vi "sm125_acquire.vi"(0 "address":string="10.0.0.212", 2 "open and close":bool=TRUE, 4 "connection ID":refnum<k5>, 5 "linear fit (PD)":bool) -> (14 "Output graph":cluster{dbl[], dbl[]}[](graph), 17 "Main Cluster":T1={"HeaderSize"=20, "Version"=1, "nChannels"=4, "freshestDut"=15, "counter"=4086}, 18 "counter":u32=4086, 19 "WvlIncrement":dbl=0.005)   [LabVIEW 2009]
uses:
  <vilib>/Analysis/NI_AALPro.lvlib
panel:
  in  "remote port":u16=50000
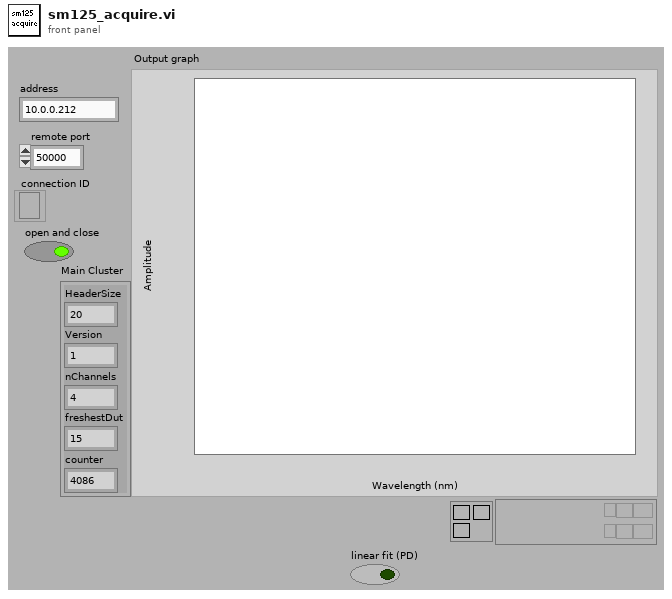
[diagram p1: front panel]
types:
  T1 = cluster{"HeaderSize":u16, "Version":u16, "nChannels":u16, "freshestDut":u16, "counter":u16}
  T2 = cluster{"HeaderSize":u16, "Version":u16, "nChannels":u16, "freshestDut":u16, "counter":i32}
  T3 = cluster{"HeaderSize":u16, "MinWvl":dbl, "WvlIncrement":dbl, "nPoints":u16, "DUT":u16}
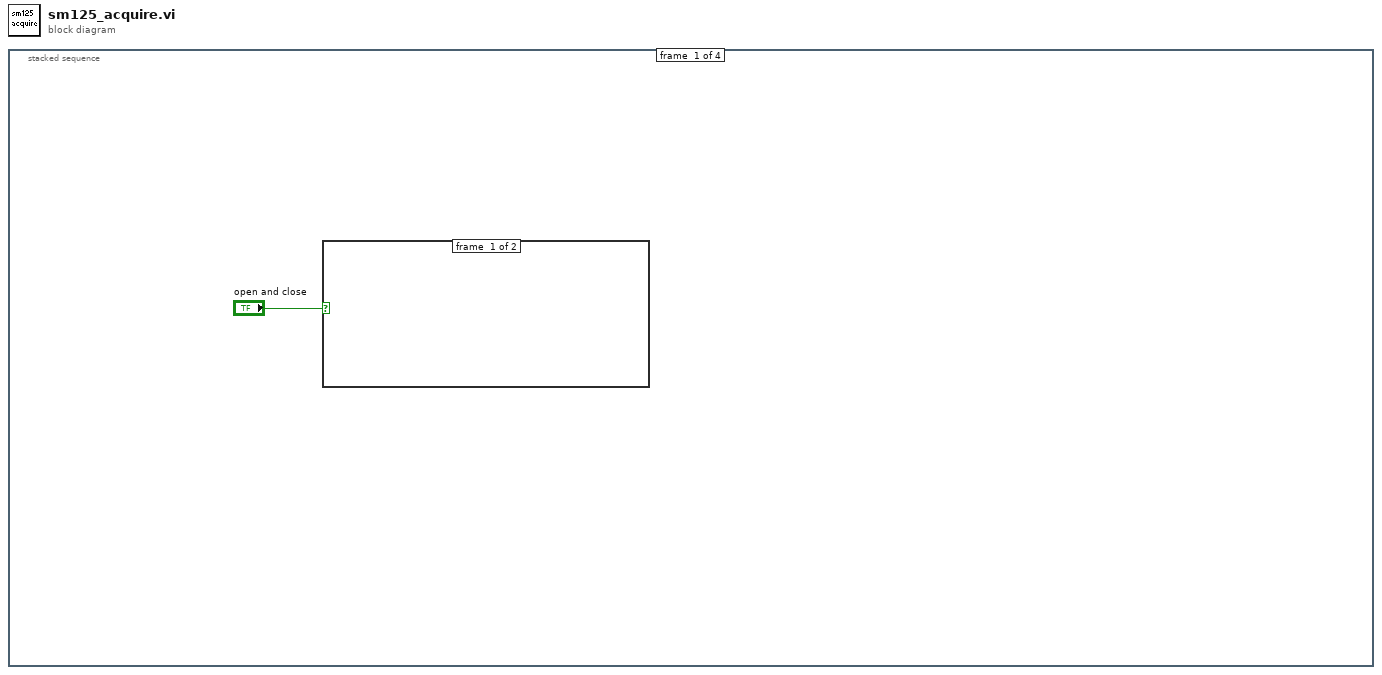
[diagram p0: block diagram]
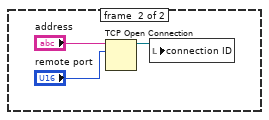
[diagram p2: hidden frame]
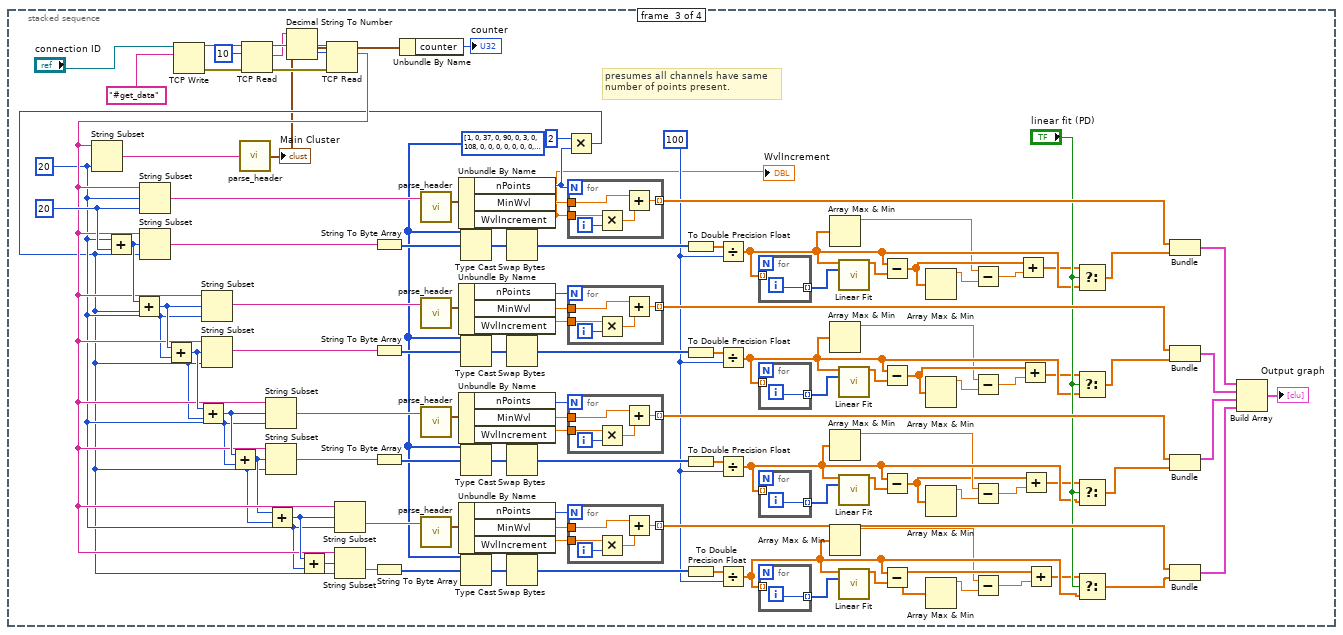
[diagram p4: hidden frame]
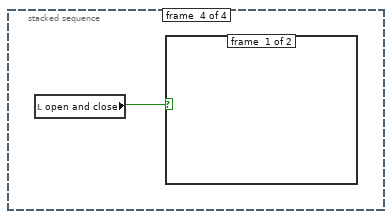
[diagram p5: hidden frame]
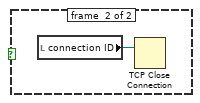
[diagram p6: hidden frame]
diagram:
  n1 = stacked-sequence {
    frame #0 {
      n2 = case shown="True" "open and close" {
        frame #0 {
        }
        frame #1 {
          n3 = TCP Open Connection(address="address", remote port or service name="remote port") -> (connection ID=w4:refnum<k5>)  [unwired: 3 in, 1 out]
          n4 = local write "connection ID"(w4) -> ()
        }
      }
    }
    frame #1 {
    }
    frame #2 {
      w56 = 100
      w57 = i16[] [1, 0, 37, 0, 90, 0, 3, 0, 108, 0, 0, 0, 0, 0, 0, 0, 0, 0, 0, 0, 0, 0, 0, 0, 0, 0, 0, 0, 0, 0, 0, 0, 0, 0, 0, 0, 0, 0, 0, 0, 0, 0, 0, 0, 0, 0, 0, 0, 0, 0, 0, 0, 0, 0, 0, 0, 0, 0, 0, 0, 0, 0, 0, 0, 32, 0, 14, 152, 140, 62, 252, 150, 1, 0, 76, 78, 0, 0, 0, 0, 0, 0, 0, 0, 0, 0, 12, 0, 0, 0, 0, 0, 0, 0, 0, 0, 0, 0, 0, 0, 0, 0, 0, 0, 0, 0, 0, 0, 0, 0, 0, 0, 0, 0, 0, 0, 0, 0, 0, 0, 0, 0, 0, 0, 0, 0, 0, 0, 92, 121, 255, 255, 0, 0, 0, 0, 0, 0, 0, 0, 0, 0, 0, 0, 0, 0, 0, 0, 0, 0, 0, 0, 0, 0, 0, 0, 0, 0, 0, 0, 0, 0, 0, 0, 0, 0, 0, 0, 0, 0, 0, 0, 0, 0, 0, 0, 0, 0, 0, 0, 0, 0, 0, 0, 0, 0, 0, 0, 0, 0, 0, 0, 82, 0, 0, 0, 0, 0, 0, 0, 0, 0, 0, 0, 0, 0, 0, 0, 0, 0, 0, 0, 0, 0, 0, 0, 0, 0, 0, 0, 0, 0, 0, 0, 0, 0, 0, 0, 0, 0, 0, 0, 0, 0, 0, 0, 0, 0, 0, 0, 0, 0, 0, 0, 0, 0, 0, 0, 0, 0, 0, 0, 0, 0, 0, 0, 110, 0, 252, 3, 183, 4, 161, 5, 181, 6, 108, 8, 117, 9, 72, 12, 25, 13, 221, 13, 76, 14, 153, 18, 218, 22, 1, 27, 14, 31, 36, 35, 56, 39, 95, 43, 152, 47, 196, 51, 8, 56, 77, 60, 162, 64, 4, 69, 115, 73, 246, 77, 121, 82, 16, 87, 171, 91, 87, 96, 4, 101, 201, 105, 146, 110, 64, 115, 24, 120, 252, 124, 229, 129, 255, 255, 255, 255, 0, 0, 0, 0, 0, 0, 0, 0, 0, 0, 0, 0, 0, 0, 0, 0, 0, 0, 0, 0, 0, 0, 0, 0, 0, 0, 0, 0, 0, 0, 0, 0, 0, 0, 0, 0, 0, 0, 0, 0, 0, 0, 0, 0, 0, 0, 0, 0, 0, 0, 0, 0, 0, 0, 0, 0, 0, 0, 0, 0, 0, 0, 0, 0, 0, 0, 0, 0, 0, 0, 0, 0, 0, 0, 0, 0, 0, 0, 0, 0, 0, 0, 0, 0, 0, 0, 0, 0, 0, 0, 0, 0, 0, 0, 0, 0, 0, 0, 0, 0, 0, 0, 0, 0, 0, 0, 0, 0, 0, 0, 0, 0, 0, 0, 0, 0, 0, 0, 0, 0, 0, 0, 0, 0, 0, 0, 0, 0, 0, 0, 0, 0, 0, 0, 0, 0, 0, 0, 0, 0, 0, 0, 0, 0, 0, 0, 0, 0, 0, 0, 0, 0, 0, 0, 0, 0, 0, 0, 0, 0, 0, 0, 0, 0, 0, 0, 0, 0, 0, 0, 0, 0, 0, 0, 0, 0, 0, 0, 77, 2, 234, 3, 164, 4, 145, 5, 168, 6, 113, 8, 131, 9, 129, 10, 107, 11, 67, 12, 5, 13, 189, 13, 109, 14, 21, 15, 205, 15, 129, 16, 33, 17, 195, 17, 99, 18, 243, 18, 151, 19, 9, 21, 154, 21, 45, 22, 192, 22, 95, 23, 190, 25, 152, 26, 155, 27, 181, 29, 50, 30, 3, 32, 38, 34, 247, 34, 253, 37, 135, 38, 249, 38, 146, 39, 127, 42, 48, 43, 60, 44, 197, 44, 47, 47, 185, 47, 72, 48, 208, 48, 210, 50, 86, 51, 195, 51, 145, 55, 36, 56, 164, 56, 102, 57, 18, 60, 129, 60, 3, 62, 120, 62, 180, 63, 168, 68, 133, 69, 106, 70, 98, 73, 82, 74, 61, 78, 7, 83, 195, 83, 164, 84, 153, 87, 25, 88, 98, 92, 90, 93, 7, 94, 3, 97, 243, 97, 220, 98, 204, 101, 186, 102, 177, 103, 182, 106, 169, 107, 84, 108, 49, 112, 149, 117, 33, 122, 22, 127, 182, 133, 240, 137, 245, 142, 47, 147, 54, 152, 255, 255, 235, 151, 199, 152, 204, 153, 155, 157, 80, 158, 190, 158, 255, 255, 255, 255, 255, 255, 31, 158, 218, 158, 255, 255, 153, 157, 255, 255, 255, 255, 255, 255, 207, 158, 238, 161, 214, 162, 255, 255, 255, 255, 0, 0, 0, 0, 0, 0, 0, 0, 0, 0, 0, 0, 0, 0, 0, 0, 0, 0, 0, 0, 0, 0, 0, 0, 0, 0, 0, 0, 0, 0, 0, 0, 59, 40, 239, 82, 166, 129, 255, 255, 255, 255, 0, 0, 0, 0, 0, 0, 0, 0, 0, 0, 0, 0, 0, 0, 0, 0, 0, 0, 0, 0, 0, 0, 0, 0, 0, 0, 0, 0, 0, 0, 0, 0, 0, 0, 0, 0, 0, 0, 0, 0, 0, 0, 0, 0, 0, 0, 0, 0, 0, 0, 0, 0, 0, 0, 0, 0, 0, 0, 0, 0, 0, 0, 0, 0, 0, 0, 0, 0, 0, 0, 0, 0, 0, 0, 0, 0, 0, 0, 0, 0, 0, 0, 0, 0, 0, 0, 0, 0, 0, 0, 0, 0, 0, 0, 0, 0, 0, 0, 0, 0, 0, 0, 0, 0, 0, 0, 0, 0, 0, 0, 0, 0, 0, 0, 0, 0, 0, 0, 0, 0, 0, 0, 0, 0, 0, 0, 0, 0, 0, 0, 0, 0, 0, 0, 0, 0, 0, 0, 0, 0, 0, 0, 0, 0, 0, 0, 0, 0, 0, 0, 0, 0, 0, 0, 0, 0, 0, 0, 0, 0, 0, 0, 0, 0, 0, 0, 0, 0, 0, 0, 0, 0, 0, 0, 0, 0, 0, 0, 0, 0, 0, 0, 0, 0, 0, 0, 0, 0, 0, 0, 0, 0, 0, 0, 0, 0, 0, 0, 0, 0, 0, 0, 0, 0, 0, 0, 0, 0, 0, 0, 0, 0, 0, 0, 0, 0, 0, 0, 0, 0, 0, 0, 0, 0, 0, 0, 0, 0, 0, 0, 0, 0, 0, 0, 0, 0, 0, 0, 0, 0, 0, 0, 0, 0, 0, 0, 93, 2, 12, 3, 214, 3, 152, 4, 117, 8, 137, 9, 122, 10, 102, 11, 66, 12, 4, 13, 150, 13, 121, 14, 37, 15, 205, 15, 115, 16, 26, 17, 188, 17, 24, 19, 180, 19, 74, 20, 224, 20, 132, 21, 36, 24, 168, 24, 50, 25, 169, 25, 173, 27, 103, 28, 159, 31, 16, 32, 149, 32, 22, 33, 165, 33, 247, 35, 131, 36, 236, 36, 173, 39, 96, 40, 209, 40, 98, 41, 205, 43, 66, 44, 208, 44, 92, 45, 197, 47, 76, 48, 213, 48, 208, 51, 150, 52, 172, 53, 164, 55, 42, 56, 165, 56, 112, 57, 127, 60, 4, 62, 26, 63, 248, 63, 125, 64, 227, 64, 189, 65, 127, 66, 123, 67, 235, 67, 157, 68, 121, 69, 82, 73, 77, 74, 78, 77, 44, 78, 254, 81, 254, 82, 173, 83, 16, 86, 188, 86, 139, 87, 139, 90, 101, 91, 57, 92, 248, 94, 251, 95, 234, 96, 239, 99, 215, 100, 181, 101, 215, 103, 190, 104, 163, 105, 176, 108, 148, 109, 83, 110, 104, 111, 84, 112, 135, 118, 18, 124, 238, 128, 217, 133, 20, 138, 246, 142, 17, 147, 41, 152, 199, 157, 215, 161, 39, 168, 182, 171, 55, 177, 245, 181, 75, 186, 255, 255, 7, 147, 150, 147, 226, 151, 195, 152, 194, 153, 207, 156, 140, 157, 75, 158, 76, 161, 202, 161, 172, 162, 190, 165, 153, 166, 148, 167, 134, 170, 68, 171, 25, 172, 10, 173, 39, 175, 255, 255, 0, 0, 0, 0, 0, 0, 0, 0, 0, 0, 0, 0, 0, 0, 0, 0, 0, 0, 0, 0, 0, 0, 0, 0, 0, 0, 0, 0, 0, 0, 0, 0, 0, 0, 0, 0, 0, 0, 0, 0, 0, 0, 0, 0, 0, 0, 0, 0, 0, 0, 0, 0, 0, 0, 0, 0, 0, 0, 0, 0, 0, 0, 0, 0, 0, 0, 0, 0, 0, 0, 0, 0, 0, 0, 0, 0, 0, 0, 0, 0, 0, 0, 0, 0, 0, 0, 0, 0, 0, 0, 0, 0, 0, 0, 0, 0, 0, 0, 0, 0, 0, 0, 0, 0, 0, 0, 0, 0, 0, 0, 0, 0, 0, 0, 0, 0, 0, 0, 0, 0, 0, 0, 0, 0, 0, 0, 0, 0, 0, 0, 0, 0, 0, 0, 0, 0, 0, 0, 0, 0, 0, 0, 0, 0, 0, 0, 0, 0, 0, 0, 0, 0, 0, 0, 0, 0, 0, 0, 0, 0, 0, 0, 0, 0, 0, 0, 0, 0, 0, 0, 0, 0, 0, 0, 0, 0, 0, 0, 0, 0, 0, 0, 0, 0, 0, 0, 0, 0, 0, 0, 0, 0, 0, 0, 0, 0, 0, 0, 0, 0, 0, 0, 0, 0, 0, 0, 0, 0, 0, 0, 0, 0, 0, 0, 0, 0, 0, 0, 0, 0, 0, 0, 0, 0, 0, 0, 0, 0, 0, 0, 0, 0, 0, 0, 0, 0, 0, 0, 0, 0, 0, 0, 0, 0, 0, 0, 0, 0, 0, 0, 0, 0, 0, 0, 85, 33, 129, 181, 194, 126, 33, 18, 52, 165, 153, 175, 177, 188, 188, 185, 180, 190, 184, 197, 191, 183, 183, 189, 186, 184, 186, 190, 190, 196, 193, 198, 199, 203, 201, 204, 203, 203, 0, 0, 0, 0, 0, 0, 0, 0, 0, 0, 0, 0, 0, 0, 0, 0, 0, 0, 0, 0, 0, 0, 0, 0, 0, 0, 0, 0, 0, 0, 0, 0, 0, 0, 0, 0, 0, 0, 0, 0, 0, 0, 0, 0, 0, 0, 0, 0, 0, 0, 0, 0, 0, 0, 0, 0, 0, 0, 0, 0, 0, 0, 0, 0, 0, 0, 0, 0, 0, 0, 0, 0, 0, 0, 0, 0, 0, 0, 0, 0, 0, 0, 0, 0, 0, 0, 0, 0, 0, 0, 65, 98, 149, 164, 162, 138, 125, 53, 132, 142, 148, 153, 154, 141, 81, 134, 124, 136, 116, 127, 89, 107, 106, 121, 121, 94, 101, 86, 96, 79, 103, 99, 105, 96, 88, 96, 88, 96, 98, 82, 94, 96, 83, 105, 95, 97, 113, 93, 84, 84, 95, 106, 83, 83, 80, 89, 90, 81, 86, 86, 78, 83, 82, 84, 90, 86, 85, 94, 83, 82, 88, 95, 99, 98, 97, 98, 107, 104, 99, 96, 92, 200, 88, 88, 87, 90, 88, 96, 88, 99, 89, 91, 101, 87, 84, 98, 94, 92, 105, 90, 85, 95, 96, 85, 95, 92, 89, 109, 112, 98, 101, 0, 0, 0, 0, 0, 0, 0, 0, 0, 0, 0, 0, 0, 0, 0, 0, 0, 23, 20, 20, 255, 0, 0, 0, 0, 0, 0, 0, 0, 0, 0, 0, 0, 0, 0, 0, 0, 0, 0, 0, 0, 0, 0, 0, 0, 0, 0, 0, 0, 0, 0, 0, 0, 0, 0, 0, 0, 0, 0, 0, 0, 0, 0, 0, 0, 0, 0, 0, 0, 0, 0, 0, 0, 0, 0, 0, 0, 0, 0, 0, 0, 0, 0, 0, 0, 0, 0, 0, 0, 0, 0, 0, 0, 0, 0, 0, 0, 0, 0, 0, 0, 0, 0, 0, 0, 0, 0, 0, 0, 0, 0, 0, 0, 0, 0, 0, 0, 0, 0, 0, 0, 0, 0, 0, 0, 0, 0, 0, 0, 0, 0, 0, 0, 0, 0, 0, 0, 0, 0, 0, 0, 0, 0, 0, 0, 102, 141, 144, 157, 141, 151, 155, 158, 163, 164, 135, 154, 169, 172, 172, 159, 158, 144, 153, 151, 145, 122, 125, 119, 125, 115, 124, 127, 107, 141, 123, 117, 123, 106, 118, 114, 125, 107, 125, 131, 107, 137, 129, 135, 129, 128, 133, 130, 111, 123, 112, 121, 137, 113, 103, 116, 100, 105, 104, 110, 107, 113, 96, 88, 121, 113, 115, 107, 104, 104, 124, 114, 108, 109, 100, 114, 109, 107, 107, 118, 127, 116, 126, 147, 122, 129, 112, 111, 123, 112, 115, 131, 178, 113, 110, 115, 112, 109, 119, 108, 125, 106, 109, 112, 110, 114, 104, 109, 115, 108, 111, 122, 117, 114, 115, 116, 115, 114, 111, 110, 110, 108, 112, 107, 107, 104, 104, 0, 0, 0, 0, 0, 0, 0, 0, 0, 0, 0, 0, 0, 0, 0, 0, 0, 0, 0, 0, 0, 0, 0, 0, 0, 0, 0, 0, 0, 0, 0, 0, 0, 0, 0, 0, 0, 0, 0, 0, 0, 0, 0, 0, 0, 0, 0, 0, 0, 0, 0, 0, 0, 0, 0, 0, 0, 0, 0, 0, 0, 0, 0, 0, 0, 0, 0, 0, 0, 0, 0, 0, 0, 0, 0, 0, 0, 0, 0, 0, 0, 0, 0, 0, 0, 0, 0, 0, 0, 0, 0, 0, 0, 0, 0, 0, 0, 0, 0, 0, 0, 0, 0, 0, 0, 0, 0, 0, 0, 0, 0, 0, 0, 0, 0, 0, 0, 0, 0, 0, 0, 0, 0, 0, 0, 0, 0, 0, 0] ("data 2")
      w109 = 20 ("length (rest)")
      w54 = 20 ("length (rest)")
      # "presumes all channels have same\nnumber of points present."
      n5 = Add(x=w54, y=w109) -> (x+y=w70:i32)
      n6 = TCP Write(connection ID="connection ID", data in="#get_data") -> (connection ID out=w116:refnum<k5>, error out=w114:errorcluster)  [unwired: 2 in, 1 out]
      n7 = TCP Read(connection ID=w116, bytes to read=10, error in (no error)=w114) -> (connection ID out=w115:refnum<k5>, data out=w111:string, error out=w113:errorcluster)  [unwired: 2 in]
      n8 = Decimal String To Number(string=w111) -> (number=w110:i32)  [unwired: 2 in, 1 out]
      n9 = TCP Read(connection ID=w115, bytes to read=w110, error in (no error)=w113) -> (data out=w64:string)  [unwired: 2 in, 2 out]
      n10 = String Subset(string=w64, length (rest)=w54) -> (substring=w48:string)  [unwired: 1 in]
      n11 = String Subset(string=w64, offset (0)=w54, length (rest)=w109) -> (substring=w102:string)
      n12 = call "parse_header.vi"("Main String"=w48) -> ("Main Cluster"=w43:T2)  [unwired: 13 in, 1 out]
      "Main Cluster" <- w43
      n13 = Unbundle By Name(w43) -> ("counter"=→"counter":i32)
      n14 = call "parse_header.vi"("Channel String"=w102) -> ("Channel Cluster"=w101:T3)  [unwired: 13 in, 1 out]
      n15 = Unbundle By Name(w101) -> ("nPoints"=w47:u16, "MinWvl"=w100:dbl, "WvlIncrement"=w44:dbl)
      "WvlIncrement" <- w44
      n16 = Multiply(x=u16 2, y=w47) -> (x*y=w45:u16)
      n17 = Add(x=w70, y=w45) -> (x+y=w69:i32)
      n18 = String Subset(string=w64, offset (0)=w70, length (rest)=w45) -> (substring=w106:string)
      n19 = Add(x=w69, y=w54) -> (x+y=w67:i32)
      n20 = Add(x=w67, y=w45) -> (x+y=w68:i32)
      n21 = String Subset(string=w64, offset (0)=w69, length (rest)=w54) -> (substring=w63:string)
      n22 = String Subset(string=w64, offset (0)=w67, length (rest)=w45) -> (substring=w62:string)
      n23 = Add(x=w68, y=w54) -> (x+y=w55:i32)
      n24 = String Subset(string=w64, offset (0)=w68, length (rest)=w54) -> (substring=w61:string)
      n25 = String Subset(string=w64, offset (0)=w55, length (rest)=w45) -> (substring=w60:string)
      n26 = Add(x=w55, y=w45) -> (x+y=w65:i32)
      n27 = Add(x=w65, y=w54) -> (x+y=w66:i32)
      n28 = String Subset(string=w64, offset (0)=w65, length (rest)=w54) -> (substring=w59:string)
      n29 = String Subset(string=w64, offset (0)=w66, length (rest)=w45) -> (substring=w58:string)
      n30 = String To Byte Array(string=w106) -> (unsigned byte array=w107:u8[])
      n31 = String To Byte Array(string=w62) -> (unsigned byte array=w90:u8[])
      n32 = String To Byte Array(string=w60) -> (unsigned byte array=w87:u8[])
      n33 = String To Byte Array(string=w58) -> (unsigned byte array=w72:u8[])
      n34 = call "parse_header.vi"("Channel String"=w63) -> ("Channel Cluster"=w93:T3)  [unwired: 13 in, 1 out]
      n35 = call "parse_header.vi"("Channel String"=w61) -> ("Channel Cluster"=w84:T3)  [unwired: 13 in, 1 out]
      n36 = call "parse_header.vi"("Channel String"=w59) -> ("Channel Cluster"=w75:T3)  [unwired: 13 in, 1 out]
      n37 = Unbundle By Name(w93) -> ("nPoints"=w94:u16, "MinWvl"=w96:dbl, "WvlIncrement"=w95:dbl)
      n38 = Unbundle By Name(w84) -> ("nPoints"=w83:u16, "MinWvl"=w81:dbl, "WvlIncrement"=w82:dbl)
      n39 = Unbundle By Name(w75) -> ("nPoints"=w76:u16, "MinWvl"=w78:dbl, "WvlIncrement"=w77:dbl)
      n40 = Type Cast(type=w57, x=w107) -> (*(type *) &x=w108:i16[])
      n41 = Type Cast(type=w57, x=w90) -> (*(type *) &x=w89:i16[])
      n42 = Type Cast(type=w57, x=w87) -> (*(type *) &x=w88:i16[])
      n43 = Type Cast(type=w57, x=w72) -> (*(type *) &x=w71:i16[])
      n44 = Swap Bytes(anything=w108) -> (byte swapped=w105:i16[])
      n45 = Swap Bytes(anything=w89) -> (byte swapped=w91:i16[])
      n46 = Swap Bytes(anything=w88) -> (byte swapped=w86:i16[])
      n47 = Swap Bytes(anything=w71) -> (byte swapped=w73:i16[])
      n48 = for {
        N: w47 -> [_]
        tunnel: w44 -> [w139]
        tunnel: w100 -> [w137]
        tunnel: [w136] -> w99 mode=indexing
        i -> [w140]
        n49 = Multiply(x=w139, y=w140) -> (x*y=w138:dbl)
        n50 = Add(x=w137, y=w138) -> (x+y=w136:dbl)
      }
      n51 = for {
        N: w94 -> [_]
        tunnel: w95 -> [w134]
        tunnel: w96 -> [w132]
        tunnel: [w131] -> w97 mode=indexing
        i -> [w135]
        n52 = Multiply(x=w134, y=w135) -> (x*y=w133:dbl)
        n53 = Add(x=w132, y=w133) -> (x+y=w131:dbl)
      }
      n54 = for {
        N: w83 -> [_]
        tunnel: w82 -> [w129]
        tunnel: w81 -> [w127]
        tunnel: [w126] -> w80 mode=indexing
        i -> [w130]
        n55 = Multiply(x=w129, y=w130) -> (x*y=w128:dbl)
        n56 = Add(x=w127, y=w128) -> (x+y=w126:dbl)
      }
      n57 = for {
        N: w76 -> [_]
        tunnel: w77 -> [w124]
        tunnel: w78 -> [w122]
        tunnel: [w121] -> w79 mode=indexing
        i -> [w125]
        n58 = Multiply(x=w124, y=w125) -> (x*y=w123:dbl)
        n59 = Add(x=w122, y=w123) -> (x+y=w121:dbl)
      }
      n60 = To Double Precision Float(number=w105) -> (double precision float=w104:dbl[])
      n61 = To Double Precision Float(number=w91) -> (double precision float=w92:dbl[])
      n62 = To Double Precision Float(number=w86) -> (double precision float=w85:dbl[])
      n63 = To Double Precision Float(number=w73) -> (double precision float=w74:dbl[])
      n64 = Divide(x=w104, y=w56) -> (x/y=w28:dbl[])
      n65 = Divide(x=w92, y=w56) -> (x/y=w27:dbl[])
      n66 = Divide(x=w85, y=w56) -> (x/y=w26:dbl[])
      n67 = Divide(x=w74, y=w56) -> (x/y=w25:dbl[])
      n68 = for {
        tunnel: w28 -> [_] mode=indexing
        tunnel: [w120] -> w41 mode=indexing
        i -> [w120]
      }
      n69 = for {
        tunnel: w27 -> [_] mode=indexing
        tunnel: [w119] -> w37 mode=indexing
        i -> [w119]
      }
      n70 = for {
        tunnel: w26 -> [_] mode=indexing
        tunnel: [w118] -> w36 mode=indexing
        i -> [w118]
      }
      n71 = for {
        tunnel: [w117] -> w31 mode=indexing
        tunnel: w25 -> [_] mode=indexing
        i -> [w117]
      }
      n72 = Array Max & Min(array=w28) -> (max value=w19:dbl)  [unwired: 3 out]
      n73 = Array Max & Min(array=w27) -> (max value=w14:dbl)  [unwired: 3 out]
      n74 = Array Max & Min(array=w26) -> (max value=w11:dbl)  [unwired: 3 out]
      n75 = Array Max & Min(array=w25) -> (max value=w6:dbl)  [unwired: 3 out]
      n76 = call <vilib>:"Linear Fit.vi"("Y"=w28, "X"=w41) -> ("Best Linear Fit"=w40:dbl[])  [unwired: 9 in, 4 out]
      n77 = call <vilib>:"Linear Fit.vi"("Y"=w27, "X"=w37) -> ("Best Linear Fit"=w38:dbl[])  [unwired: 9 in, 4 out]
      n78 = call <vilib>:"Linear Fit.vi"("Y"=w26, "X"=w36) -> ("Best Linear Fit"=w35:dbl[])  [unwired: 9 in, 4 out]
      n79 = call <vilib>:"Linear Fit.vi"("Y"=w25, "X"=w31) -> ("Best Linear Fit"=w32:dbl[])  [unwired: 9 in, 4 out]
      n80 = Subtract(x=w28, y=w40) -> (x-y=w20:dbl[])
      n81 = Subtract(x=w27, y=w38) -> (x-y=w15:dbl[])
      n82 = Subtract(x=w26, y=w35) -> (x-y=w10:dbl[])
      n83 = Subtract(x=w25, y=w32) -> (x-y=w7:dbl[])
      n84 = Array Max & Min(array=w20) -> (max value=w18:dbl)  [unwired: 3 out]
      n85 = Array Max & Min(array=w15) -> (max value=w16:dbl)  [unwired: 3 out]
      n86 = Array Max & Min(array=w10) -> (max value=w12:dbl)  [unwired: 3 out]
      n87 = Array Max & Min(array=w7) -> (max value=w8:dbl)  [unwired: 3 out]
      n88 = Subtract(x=w19, y=w18) -> (x-y=w17:dbl)
      n89 = Subtract(x=w14, y=w16) -> (x-y=w13:dbl)
      n90 = Subtract(x=w11, y=w12) -> (x-y=w9:dbl)
      n91 = Subtract(x=w6, y=w8) -> (x-y=w5:dbl)
      n92 = Add(x=w20, y=w17) -> (x+y=w24:dbl[])
      n93 = Add(x=w15, y=w13) -> (x+y=w23:dbl[])
      n94 = Add(x=w10, y=w9) -> (x+y=w22:dbl[])
      n95 = Add(x=w7, y=w5) -> (x+y=w21:dbl[])
      n96 = Select(t=w24, s="linear fit (PD)", f=w28) -> (s? t:f=w39:dbl[])
      n97 = Select(t=w23, s="linear fit (PD)", f=w27) -> (s? t:f=w34:dbl[])
      n98 = Select(t=w22, s="linear fit (PD)", f=w26) -> (s? t:f=w33:dbl[])
      n99 = Select(t=w21, s="linear fit (PD)", f=w25) -> (s? t:f=w30:dbl[])
      n100 = Bundle(w99, w39) -> (w98:cluster{dbl[], dbl[]})  [unwired: 1 in]
      n101 = Bundle(w97, w34) -> (w52:cluster{dbl[], dbl[]})  [unwired: 1 in]
      n102 = Bundle(w80, w33) -> (w51:cluster{dbl[], dbl[]})  [unwired: 1 in]
      n103 = Bundle(w79, w30) -> (w50:cluster{dbl[], dbl[]})  [unwired: 1 in]
      n104 = Build Array(w98, w52, w51, w50) -> (→"Output graph":cluster{dbl[], dbl[]}[])
    }
    frame #3 {
      n105 = local read "open and close"() -> (w141:bool)
      n106 = case shown="True" w141 {
        frame #0 {
        }
        frame #1 {
          n107 = local read "connection ID"() -> (w142:refnum<k5>)
          n108 = TCP Close Connection(connection ID=w142) -> ()  [unwired: 2 in, 2 out]
        }
      }
    }
  }
